vi "Set configuration chain.vi"(8 "error in (no error)":errorcluster, 9 "class names":string[](array[string]), 10 "configuration":variant[](array[variant]), 11 "ExampleClassB in":refnum<class "ExampleClassB.lvclass">) -> (0 "error out":errorcluster, 3 "ExampleClassB out":refnum<class "ExampleClassB.lvclass">)   [LabVIEW 2012, in "ExampleClassB.lvclass"]
uses:
  ExampleClassB.lvclass
  ExampleClassB.lvclass/ExampleClassB.ctl
  <vilib>/Distrio/Murmex/Murmex/Murmex.lvclass
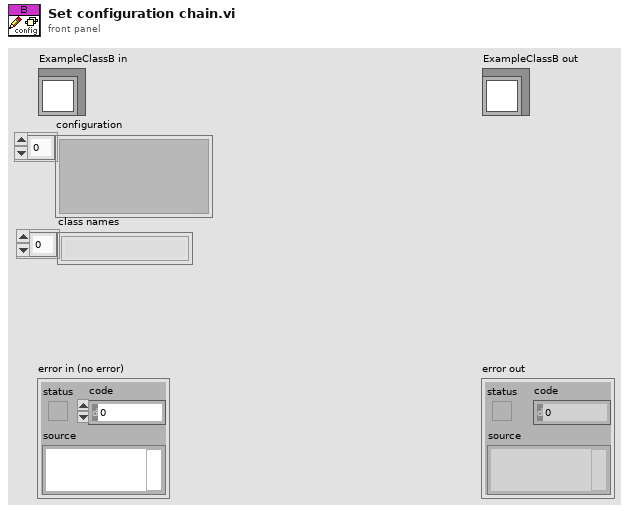
[diagram p1: front panel]
types:
  T1 = typedef "ExampleClassB.lvclass/Configuration cluster.ctl" = cluster{"scaling factor":dbl, "offset":dbl}
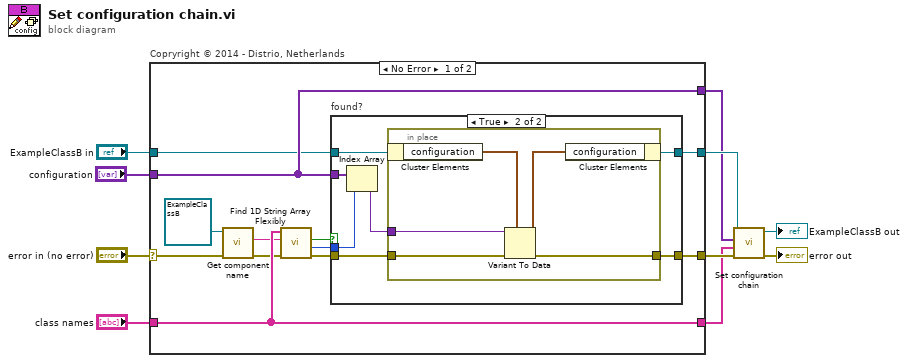
[diagram p0: block diagram]
diagram:
  n1 = case "Copryright © 2014 - Distrio, Netherlands" shown="No Error" "error in (no error)" {
    selector: "error in (no error)" -> [w22 w40]
    tunnel: [w20 w40] -> w6
    tunnel: [w21 w39] -> w5
    tunnel: "ExampleClassB in" -> [w12 w39]
    tunnel: "class names" -> [w18 w37]
    tunnel: "configuration" -> [w19 w38]
    tunnel: [w19 w38] -> w2
    tunnel: [w18 w37] -> w1
    frame No Error {
      n2 = call <vilib>:"Get component name.vi"("error in (no error)"=w22, "Murmex in"=refnum<class "ExampleClassB.lvclass"> refnum ("ExampleClassB in")) -> ("error out"=w16:errorcluster, "component name"=w17:string)  [unwired: 7 in, 1 out]
      n3 = call <vilib>:"Find 1D String Array Flexibly.vi"("error in (no error)"=w16, "element"=w17, "array"=w18) -> ("error out"=w15:errorcluster, "index of element"=w14:i32, "found?"=w13:bool)  [unwired: 6 in]
      n4 = case "found?" shown="True" w13 {
        tunnel: w12 -> [w23 w30]
        tunnel: [w23 w29] -> w21
        tunnel: [w24 w28] -> w20
        tunnel: w19 -> [_ w27]
        tunnel: w15 -> [w24 w26]
        tunnel: w14 -> [_ w25]
        frame False {
        }
        frame True {
          n5 = Index Array(array=w27, index=w25) -> (element=w31:variant)
          n6 = in-place {
            in-place-border: w31 -> [w36]
            in-place-border: w26 -> [w34]
            in-place-border: [w32] -> w28
            n7 = in-place-cluster #1(w30) -> ("configuration"=w35:T1)
            n8 = Variant To Data(error in=w34, type=w35, Variant=w36) -> (data=w33:T1, error out=w32:errorcluster)
            n9 = in-place-cluster #1("configuration"=w33) -> (w29:refnum<class "ExampleClassB.lvclass">)
          }
        }
      }
    }
    frame Error {
    }
  }
  n10 = call-parent "Set configuration chain.vi"("error in (no error)"=w6, "class names"=w1, "configuration"=w2, "Murmex in"=w5) -> ("error out"=→"error out":errorcluster, "Murmex out"=→"ExampleClassB out":refnum<class "ExampleClassB.lvclass">)  [unwired: 6 in]
